vi "Create_pop_arrays.vi"(10 "Normalized I in":dbl[](array[numeric]), 11 "Saturation Polarization":dbl) -> (1 "rho- array out":dbl[](array[numeric]), 2 "rho0 array out":dbl[](array[numeric]), 3 "rho+ array out":dbl[](array[numeric]))   [LabVIEW 2018]
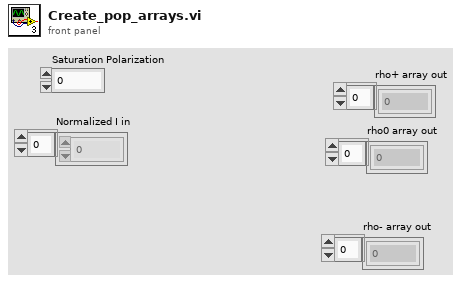
[diagram p1: front panel]
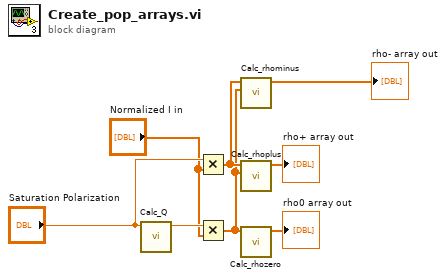
[diagram p0: block diagram]
diagram:
  n1 = call "Calc_Q.vi"("P"="Saturation Polarization") -> ("Q"=w3:dbl)  [unwired: 10 in]
  n2 = Multiply(x="Saturation Polarization", y="Normalized I in") -> (x*y=w5:dbl[])
  n3 = Multiply(x=w3, y="Normalized I in") -> (x*y=w4:dbl[])
  n4 = call "Calc_rhominus.vi"("Q"=w4, "P"=w5) -> ("rho+"=→"rho- array out":dbl[])  [unwired: 9 in]
  n5 = call "Calc_rhoplus.vi"("Q"=w4, "P"=w5) -> ("rho+"=→"rho+ array out":dbl[])  [unwired: 9 in]
  n6 = call "Calc_rhozero.vi"("Q"=w4) -> ("rho+"=→"rho0 array out":dbl[])  [unwired: 9 in]
